vi "Urgency Comparison.vi"(8 "SR Cluster 2 in":T1 {"Creation Date" format="%<%x>T"; "Last Updated" format="%<%x>T"}, 9 "SR Cluster 1 in":T1 {"Creation Date" format="%<%x>T"; "Last Updated" format="%<%x>T"}, 10 "flip? in":bool, 11 "equal? in":bool) -> (0 "SR Cluster 2 out":T1 {"Creation Date" format="%<%x>T"; "Last Updated" format="%<%x>T"}, 1 "SR Cluster 1 out":T1 {"Creation Date" format="%<%x>T"; "Last Updated" format="%<%x>T"}, 2 "flip? out":bool, 3 "equal? out":bool)   [LabVIEW 2018]
uses:
  Type Defs/SR Cluster.ctl
  Type Defs/SR Status.ctl
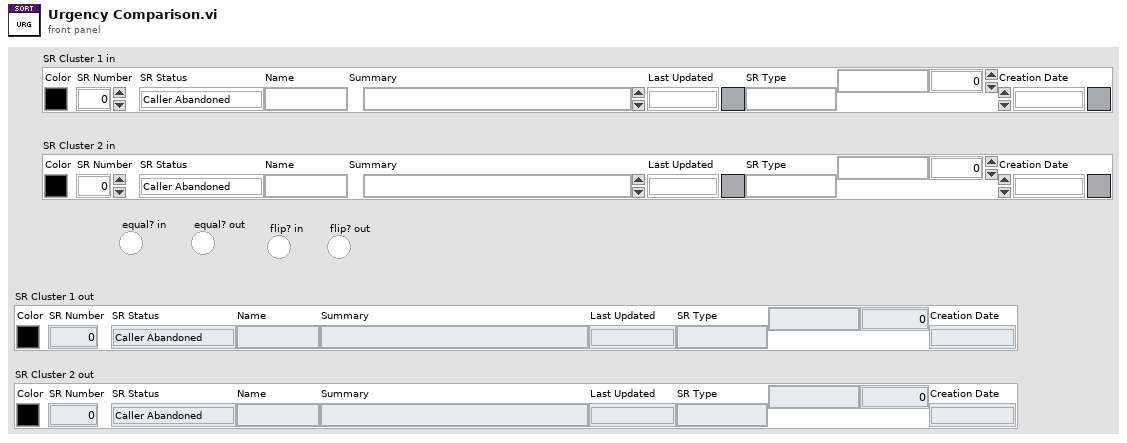
[diagram p1: front panel]
types:
  T1 = typedef "SR Cluster.ctl" = cluster{"Color":u32, "SR Number":i32, "SR Status":T2, "Name":string, "Summary":string, "Last Updated":timestamp, "SR Type":string, "Service Level":string, "Days Open":dbl, "Creation Date":timestamp}
  T2 = typedef "SR Status.ctl" = enum16{"Caller Abandoned", "Created in Error", "Expired", "Forum Resolved AE", "Forum Resolved Customer", "IN WORK", "IN WORK Collab with AES", "IN WORK Collab with PSE", "IN WORK Collab with SE", "IN WORK Customer Added Note", "IN WORK Escalation", "IN WORK Wait on Customer", "Open", "Potentially Resolved", "Presumed Resolved", "RMA Approved for Return", "RMA Closed", "RMA Closed - DOA", "RMA In Progress", "RMA Open", "RMA Waiting on Customer", "Resolved", "Passed Off"}
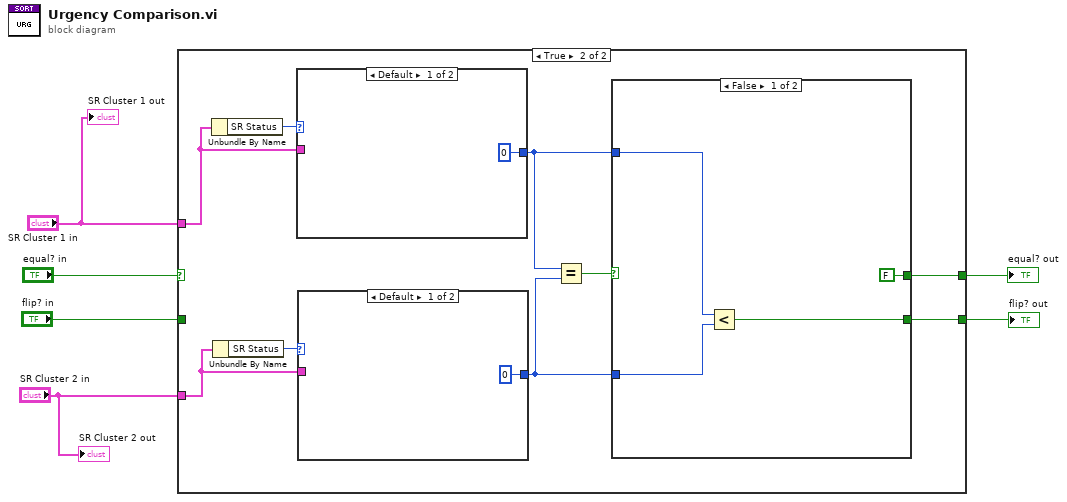
[diagram p0: block diagram]
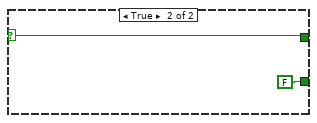
[diagram p3: hidden frame]
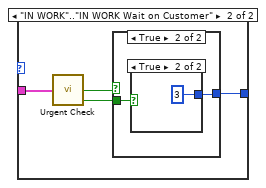
[diagram p4: hidden frame]
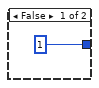
[diagram p5: hidden frame]
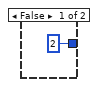
[diagram p6: hidden frame]
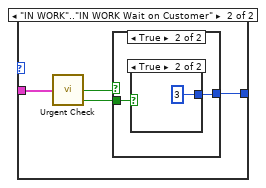
[diagram p7: hidden frame]
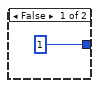
[diagram p8: hidden frame]
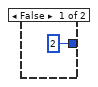
[diagram p9: hidden frame]
diagram:
  n1 = case shown="True" "equal? in" {
    selector: "equal? in" -> [w7 _]
    tunnel: [w8 w11] -> w6
    tunnel: "flip? in" -> [w8 _]
    tunnel: [w7 w12] -> w3
    tunnel: "SR Cluster 2 in" -> [_ w14]
    tunnel: "SR Cluster 1 in" -> [_ w17]
    frame False {
    }
    frame True {
      n2 = Unbundle By Name(w17) -> ("SR Status"=w16:T2)
      n3 = Unbundle By Name(w14) -> ("SR Status"=w15:T2)
      n4 = case shown="Default" w16 {
        tunnel: w17 -> [_ w38]
        tunnel: [0 w35] -> w10
        frame Default {
        }
        frame "IN WORK".."IN WORK Wait on Customer" {
          n5 = call "Urgent Check.vi"("SR Cluster"=w38) -> ("Passed Due?"=w36:bool, "Answer Today?"=w37:bool)  [unwired: 3 in]
          n6 = case shown="True" w37 {
            tunnel: w36 -> [_ w41]
            tunnel: [1 w40] -> w35
            frame False {
            }
            frame True {
              n7 = case shown="True" w41 {
                tunnel: [2 3] -> w40
                frame False {
                }
                frame True {
                }
              }
            }
          }
        }
      }
      n8 = case shown="Default" w15 {
        tunnel: w14 -> [_ w28]
        tunnel: [0 w25] -> w9
        frame Default {
        }
        frame "IN WORK".."IN WORK Wait on Customer" {
          n9 = call "Urgent Check.vi"("SR Cluster"=w28) -> ("Passed Due?"=w26:bool, "Answer Today?"=w27:bool)  [unwired: 3 in]
          n10 = case shown="True" w27 {
            tunnel: w26 -> [_ w31]
            tunnel: [1 w30] -> w25
            frame False {
            }
            frame True {
              n11 = case shown="True" w31 {
                tunnel: [2 3] -> w30
                frame False {
                }
                frame True {
                }
              }
            }
          }
        }
      }
      n12 = Equal?(x=w10, y=w9) -> (x = y?=w13:bool)
      n13 = case shown="False" w13 {
        selector: w13 -> [_ w22]
        tunnel: [FALSE w22] -> w12
        tunnel: [w19 FALSE] -> w11
        tunnel: w10 -> [w21 _]
        tunnel: w9 -> [w20 _]
        frame False {
          n14 = Less?(x=w21, y=w20) -> (x < y?=w19:bool)
        }
        frame True {
        }
      }
    }
  }
  "equal? out" <- w3
  "flip? out" <- w6
  "SR Cluster 2 out" <- "SR Cluster 2 in"
  "SR Cluster 1 out" <- "SR Cluster 1 in"
